vi "4000_Strip_Checksum.vi"(5 "ADAM response":string) -> (0 "Comment out":string, 2 "ADAM reading":string)   [LabVIEW 2010]
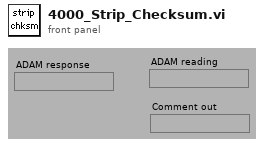
[diagram p1: front panel]
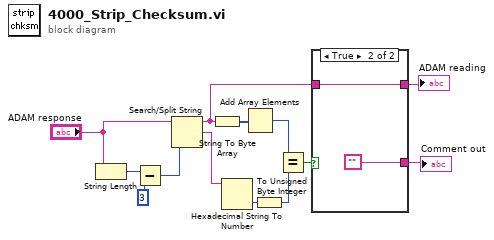
[diagram p0: block diagram]
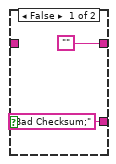
[diagram p2: hidden frame]
diagram:
  n1 = String Length(string="ADAM response") -> (length=w5:i32)
  n2 = Subtract(x=w5, y=3) -> (x-y=w7:i32)
  n3 = Search/Split String(string="ADAM response", offset (0)=w7) -> (substring before match=w1:string, match + rest of string=w10:string)  [unwired: 2 out]
  n4 = String To Byte Array(string=w1) -> (unsigned byte array=w8:u8[])
  n5 = Hexadecimal String To Number(string=w10) -> (number=w12:u32)  [unwired: 3 out]
  n6 = Add Array Elements(numeric array=w8) -> (sum=w11:u8)
  n7 = To Unsigned Byte Integer(number=w12) -> (unsigned 8bit integer=w13:u8)
  n8 = Equal?(x=w11, y=w13) -> (x = y?=w4:bool)
  n9 = case shown="True" w4 {
    tunnel: ["Bad Checksum;" ("false string") ""] -> w3
    tunnel: ["" w16] -> w2
    tunnel: w1 -> [_ w16]
    frame False {
    }
    frame True {
    }
  }
  "ADAM reading" <- w2
  "Comment out" <- w3
